vi "Simple TCP - Client_Modified.vi"() -> ()   [LabVIEW 2020]
doc: "Demonstrates how to open a connection to an TCP server, read the data being sent, and display the data on a chart. This VI is designed to stop if the TCP connection is terminated."
panel:
  out "data out":string="Bad Password\r\n"
  in  "Server Closed":string="The server VI closed the connection."
  in  "Stop":bool
  # "Overview: Demonstrates the use of the TCP functions to connect to a TCP server VI and receive data.\nInstructions:\n1. Ensure Simple TCP - Server.vi is already running.\n2. Run the VI.\n3. Click Stop to stop the VI. Note that if you stop the server VI, this VI will stop automatically."
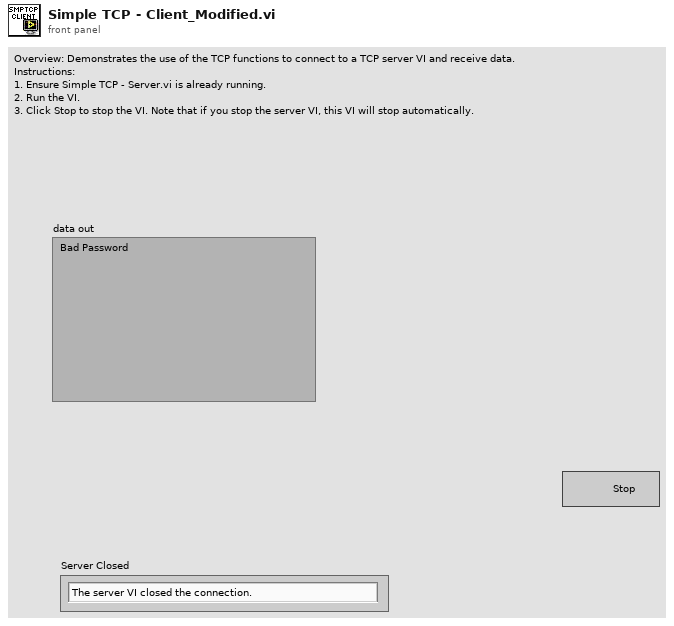
[diagram p1: front panel]
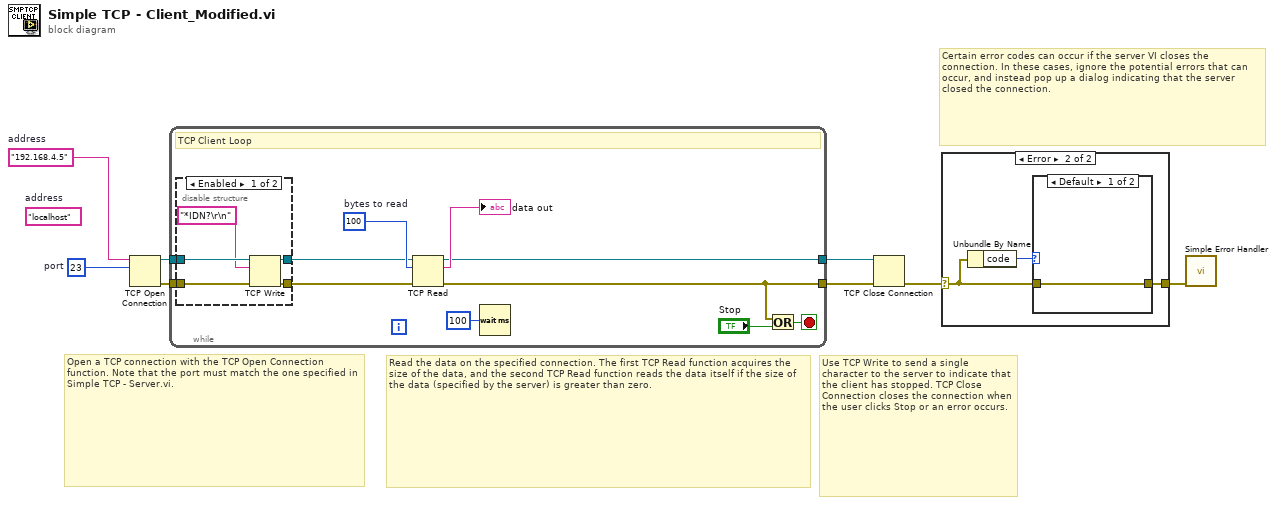
[diagram p0: block diagram]
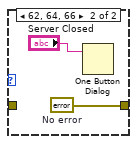
[diagram p3: hidden frame]
diagram:
  w3 = "192.168.4.5"  # address
  w4 = u16 23  # port
  (unwired) "localhost"  # address
  # "Certain error codes can occur if the server VI closes the connection. In these cases, ignore the potential errors that can occur, and instead pop up a dialog indicating that the server closed the connection."
  # "Use TCP Write to send a single character to the server to indicate that the client has stopped. TCP Close Connection closes the connection when the user clicks Stop or an error occurs."
  # "Read the data on the specified connection. The first TCP Read function acquires the size of the data, and the second TCP Read function reads the data itself if the size of the data (specified by the server) is greater than zero."
  # "Open a TCP connection with the TCP Open Connection function. Note that the port must match the one specified in Simple TCP - Server.vi."
  n1 = TCP Open Connection(address=w3, remote port or service name=w4) -> (connection ID=w8:refnum<k5>, error out=w7:errorcluster)  [unwired: 3 in]
  n2 = while {
    tunnel: w7 -> [w11]
    tunnel: w8 -> [w9]
    tunnel: [w14] -> w2
    tunnel: [w13] -> w1
    stop <- w16 stop-if-true
    w18 = 100  # bytes to read
    # "TCP Client Loop"
    n3 = disable-structure shown="Enabled" {
      disable-tunnel: [w24 w25] -> w12
      disable-tunnel: w11 -> [w23 w25]
      disable-tunnel: [w22 w26] -> w10
      disable-tunnel: w9 -> [w21 w26]
      frame Enabled {
        n4 = TCP Write(connection ID=w21, data in="*IDN?\r\n", error in (no error)=w23) -> (connection ID out=w22:refnum<k5>, error out=w24:errorcluster)  [unwired: 1 in, 1 out]
      }
      frame Disabled {
      }
    }
    n5 = TCP Read(connection ID=w10, bytes to read=w18, error in (no error)=w12) -> (connection ID out=w14:refnum<k5>, data out=→"data out":string, error out=w13:errorcluster)  [unwired: 2 in]
    n6 = Wait (ms)(milliseconds to wait=u32 100) -> ()  [unwired: 1 out]
    n7 = Or(x=w13, y="Stop") -> (x .or. y?=w16:bool)
  }
  n8 = TCP Close Connection(connection ID=w2, error in (no error)=w1) -> (error out=w6:errorcluster)  [unwired: 1 in, 1 out]
  n9 = case shown="Error" w6 {
    selector: w6 -> [w27 w29]
    tunnel: [w27 w28] -> w5
    frame No Error {
    }
    frame Error {
      n10 = Unbundle By Name(w29) -> ("code"=w30:i32)
      n11 = case shown="Default" w30 {
        tunnel: w29 -> [w31 _]
        tunnel: [w31 w33] -> w28
        frame Default {
        }
        frame 62, 64, 66 {
          w33 = errorcluster {"status"=FALSE, "code"=0, "source"=""}  # No error
          n12 = One Button Dialog(message="Server Closed") -> ()  [unwired: 1 in, 1 out]
        }
      }
    }
  }
  n13 = call <vilib>:"Simple Error Handler.vi"("error in (no error)"=w5) -> ()  [unwired: 4 in, 5 out]
